vi "from string.vi"(8 "error in":errorcluster, 9 "data":string, 10 "version":string, 11 "fixed channel configuration in":refnum<class "ThreePhasePLL configuration.lvclass">) -> (0 "error out":errorcluster, 3 "fixed channel configuration out":refnum<class "ThreePhasePLL configuration.lvclass">)   [LabVIEW 2017, in "ThreePhasePLL configuration.lvclass"]
doc: "Provides an interface for loading a module configuration from a file or other serialized data source. It is recommended that all children of this class store data in two sets--data required for its own initialization, and any data required for parent initialization--and that each implementation uses the <b>Call Parent Method</b> primitive to de-serialize parent information. As a result, it is expected that every module configuration class calls <b>component configuration.lvclass:From String.vi</b>.\nNI Tag Bus Module Framework 1.0.3.43\nNI Systems Engineering"
uses:
  ThreePhasePLL configuration.lvclass
  <vilib>/NI/PowerElectronicsControl/ThreePhasePLL/Interface/Configuration.ctl
  <vilib>/rvi/Analysis/control/PID/Typedef/niFpgaPID_PIGains.ctl
  <vilib>/rvi/Analysis/control/PID/Typedef/niFpgaPID_OutputRange.ctl
  ThreePhasePLL configuration.lvclass/ThreePhasePLL configuration.ctl
  <vilib>/NI/DCAF/Tag Editor Core/control module/configuration/control module configuration.lvclass
  <vilib>/NI/Configuration Framework/serializable configuration/NISE_CEF_serializable configuration.lvclass
  <vilib>/NI/PowerElectronicsControl/ThreePhasePLL/Interface/ThreePhasePLLInterface.lvlib
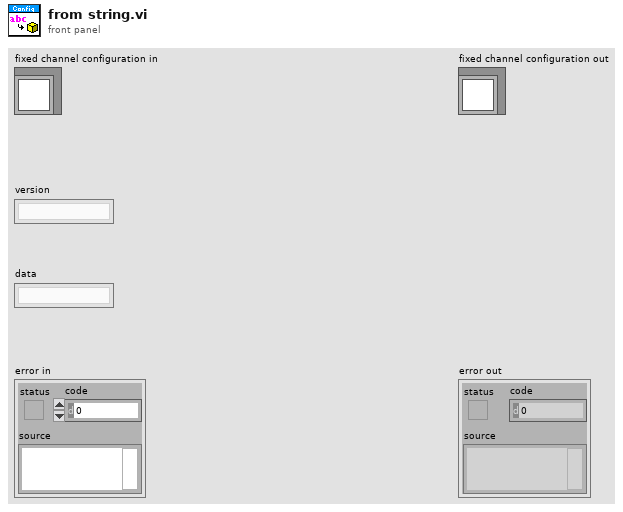
[diagram p1: front panel]
types:
  T1 = typedef "ThreePhasePLLInterface.lvlib/Configuration.ctl" = cluster{"PLLgains":T2, "PLLrange":T3, "dT":sgl, "expectedFreq":sgl, "lockDuration":sgl, "freqBoundaries":sgl}
  T2 = typedef "niFpgaPID_PIGains.ctl" = cluster{"proportional gain":sgl, "integral gain":sgl}
  T3 = typedef "niFpgaPID_OutputRange.ctl" = cluster{"output high (Inf)":sgl, "output low (-Inf)":sgl}
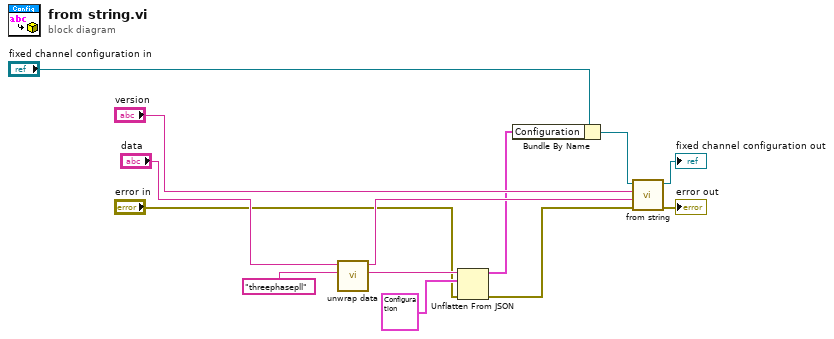
[diagram p0: block diagram]
diagram:
  n1 = call <vilib>:"unwrap data.vi"("identifier"="threephasepll", "data to unwrap"="data") -> ("unwrapped data"=w7:string, "remaining string"=w8:string)  [unwired: 8 in]
  n2 = Unflatten From JSON(JSON string=w7, type and defaults=T1 {"PLLgains"={"proportional gain"=0.0, "integral gain"=0.0}, "PLLrange"={"output high (Inf)"=inf, "output low (-Inf)"=-inf}, "dT"=0.0, "expectedFreq"=0.0, "lockDuration"=0.0, "freqBoundaries"=0.0} ("Configuration"), error in (no error)="error in") -> (value=w5:T1, error out=w1:errorcluster)  [unwired: 4 in]
  n3 = Bundle By Name(cluster="fixed channel configuration in", "Configuration"=w5) -> (w3:refnum<class "ThreePhasePLL configuration.lvclass">)
  n4 = call-parent "from string.vi"("error in"=w1, "data"=w8, "version"="version", "fixed channel configuration in"=w3) -> ("error out"=→"error out":errorcluster, "fixed channel configuration out"=→"fixed channel configuration out":refnum<class "ThreePhasePLL configuration.lvclass">)  [unwired: 6 in]
